vi "To JSON String.vi"(8 "error in (no error)":errorcluster, 11 "JSONable in":refnum<class "JSONable.lvclass">) -> (0 "error out":errorcluster, 2 "JSON String":string, 3 "JSONable out":refnum<class "JSONable.lvclass">)   [LabVIEW 2015, in "JSONable.lvclass"]
uses:
  JSONable.lvclass
  <vilib>/NI/JSON Support for LabVIEW/JSON Data Classes/JSON Datatype/JSON Null.lvclass
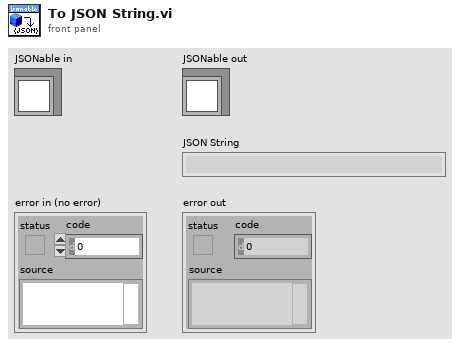
[diagram p1: front panel]
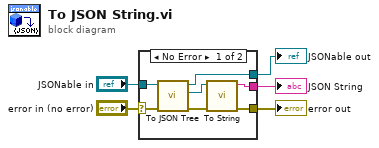
[diagram p0: block diagram]
diagram:
  n1 = case shown="No Error" "error in (no error)" {
    selector: "error in (no error)" -> [w11 w14]
    tunnel: [w7 w14] -> w4
    tunnel: [w10 w13] -> w2
    tunnel: "JSONable in" -> [w12 w13]
    tunnel: [w8 _] -> w1
    frame No Error {
      n2 = call-dynamic "To JSON Tree.vi"("error in (no error)"=w11, "JSONable in"=w12) -> ("error out"=w6:errorcluster, "JSON out"=w9:refnum<class "JSON Null.lvclass">, "JSONable out"=w10:refnum<class "JSONable.lvclass">)  [unwired: 7 in]
      n3 = call-dynamic "To String.vi"("error in (no error)"=w6, "JSON Datatype in"=w9) -> ("error out"=w7:errorcluster, "String"=w8:string)  [unwired: 8 in]
    }
    frame Error {
    }
  }
  "error out" <- w4
  "JSONable out" <- w2
  "JSON String" <- w1
